vi "VI Input Panel Resize.vi"(8 "error in (no error)":errorcluster, 10 "Input Array":refnum<vi>, 11 "Pane Ref":refnum<vi>) -> (0 "error out":errorcluster)   [LabVIEW 2015, in "CallVIStep.lvclass"]
uses:
  CallVIStep.lvclass
  <vilib>/Utility/miscctls.llb/LVPointTypeDef.ctl
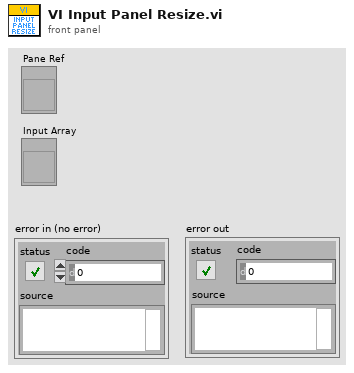
[diagram p1: front panel]
types:
  T1 = typedef "LVPointTypeDef.ctl" = cluster{"Horizontal":i16, "Vertical":i16}
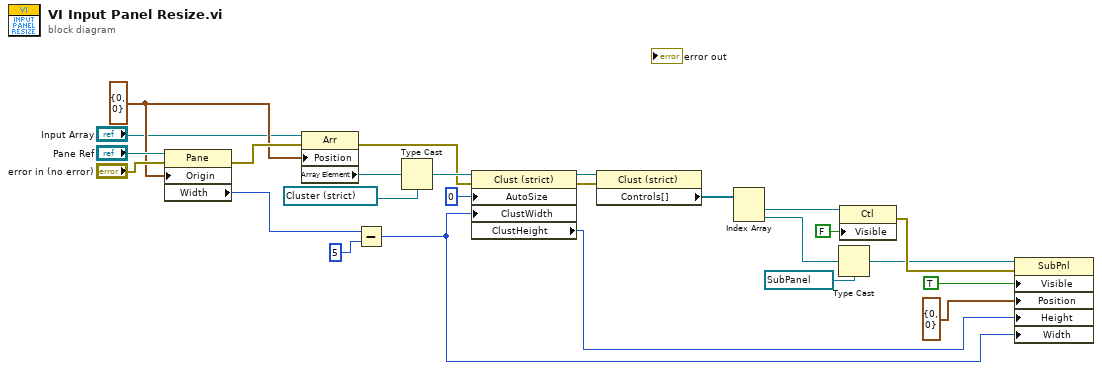
[diagram p0: block diagram]
diagram:
  w22 = T1 {"Horizontal"=0, "Vertical"=0} ("Origin")
  n1 = property class="Pane"(reference="Pane Ref", error in="error in (no error)", "Origin"=w22) -> (error out=w23:errorcluster, "Width"=w17:u32)  [unwired: 1 out]
  n2 = property class="Arr"(reference="Input Array", error in=w23, "Position"=w22) -> (error out=w19:errorcluster, "Array Element"=w21:refnum<vi>)  [unwired: 1 out]
  n3 = Subtract(x=w17, y=u32 5) -> (x-y=w2:u32)
  n4 = Type Cast(type=refnum<vi> refnum ("reference"), x=w21) -> (*(type *) &x=w20:refnum<vi>)
  n5 = property class="Clust (strict)"(reference=w20, error in=w19, "AutoSize"=u32 0 ("Auto Sizing"), "ClustWidth"=w2) -> (reference out=w3:refnum<vi>, error out=w4:errorcluster, "ClustHeight"=w1:u32)
  n6 = property class="Clust (strict)"(reference=w3, error in=w4) -> ("Controls[]"=w13:refnum<vi>[])  [unwired: 2 out]
  n7 = Index Array(array=w13) -> (element #1=w10:refnum<vi>, element #2=w8:refnum<vi>)  [unwired: 2 in]
  n8 = Type Cast(type=refnum<vi> refnum ("element"), x=w8) -> (*(type *) &x=w7:refnum<vi>)
  n9 = property class="Ctl"(reference=w10, "Visible"=FALSE) -> (error out=w9:errorcluster)  [unwired: 1 in, 1 out]
  n10 = property class="SubPnl"(reference=w7, error in=w9, "Visible"=TRUE, "Position"=T1 {"Horizontal"=0, "Vertical"=0} ("Origin"), "Height"=w1, "Width"=w2) -> ()  [unwired: 2 out]
